vi "Convert Model.vi"(3 "error in (no error)":errorcluster, 4 "Model":string, 5 "Model Name In":T1) -> (0 "error out":errorcluster, 1 "SingleSource":bool, 2 "Model Name  Out":T1)   [LabVIEW 2018]
uses:
  Type Defs/Instrument Model.ctl
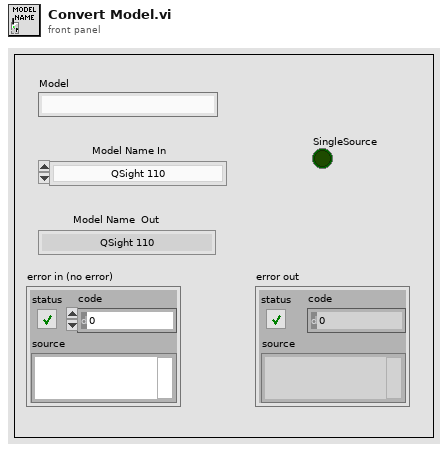
[diagram p1: front panel]
types:
  T1 = typedef "Instrument Model.ctl" = enum16{"QSight 110", "QSight 120", "QSight 210", "QSight 220", "QSight 410", "QSight 420", "IONICS 3Q 110", "IONICS 3Q 120", "IONICS 3Q 210", "IONICS 3Q 220", "IONICS 3Q 310", "IONICS 3Q 320", "Simulation (Single Source)", "Simulation (Dual Source)"}
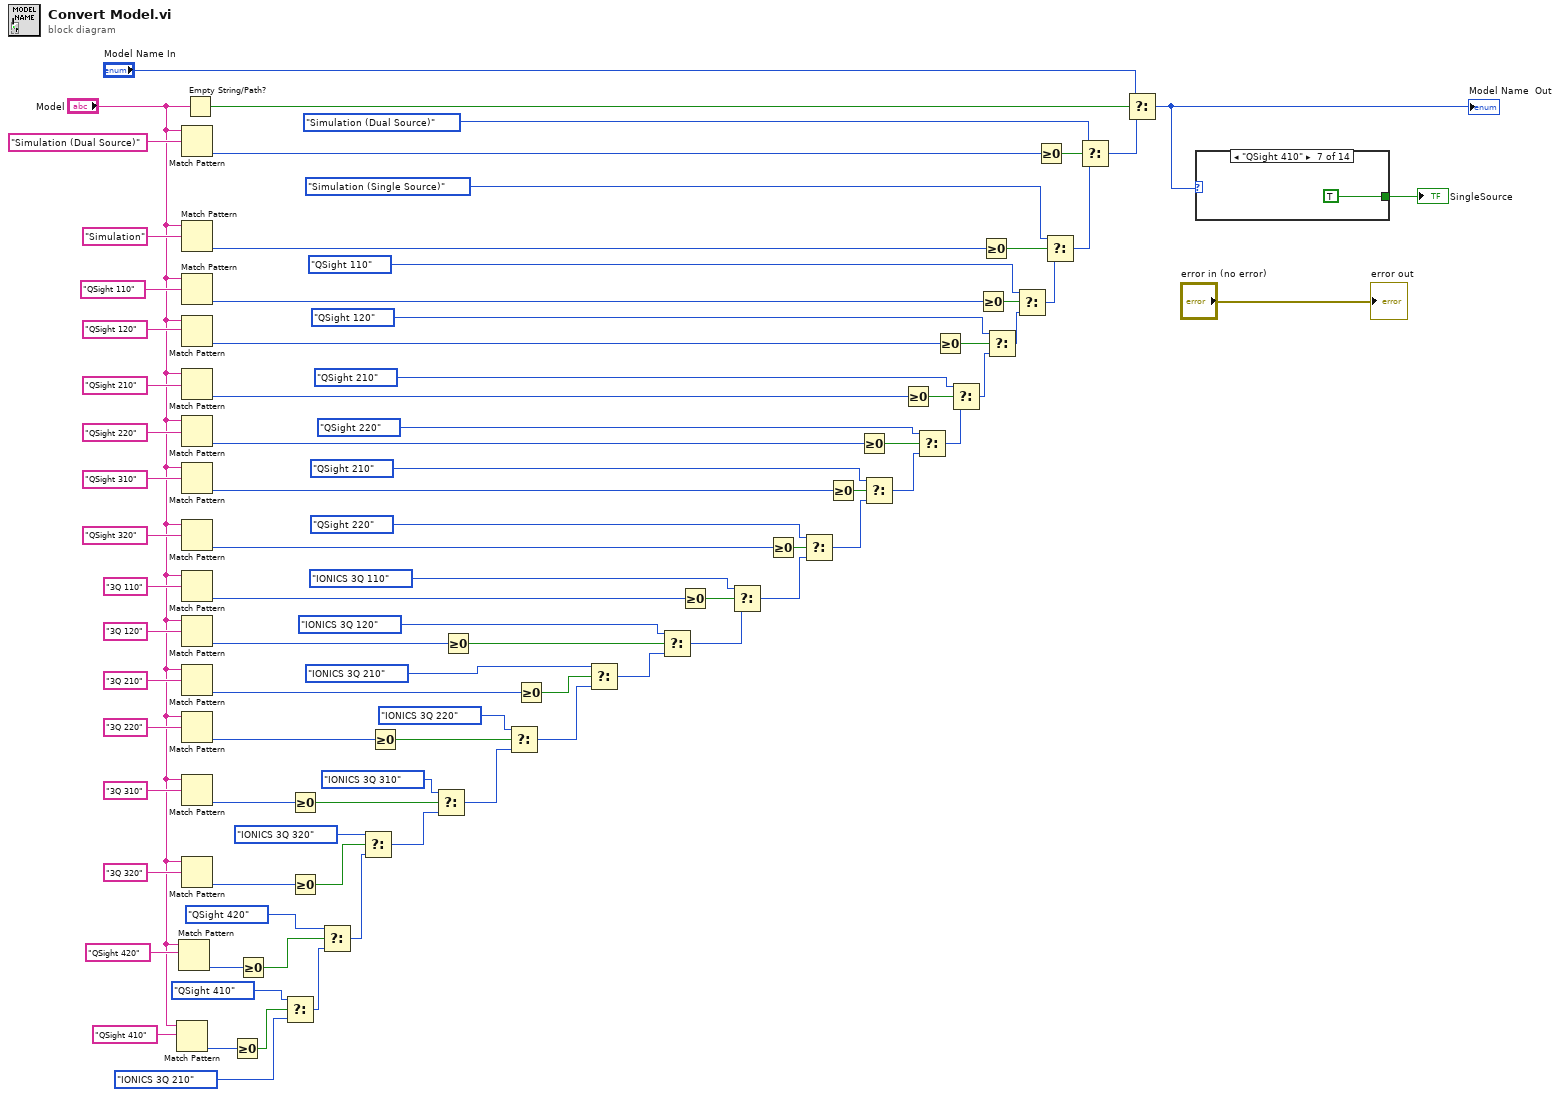
[diagram p0: block diagram]
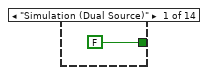
[diagram p2: hidden frame]
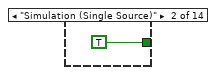
[diagram p3: hidden frame]
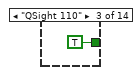
[diagram p4: hidden frame]
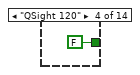
[diagram p5: hidden frame]
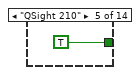
[diagram p6: hidden frame]
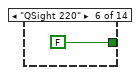
[diagram p7: hidden frame]
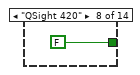
[diagram p8: hidden frame]
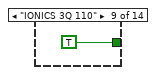
[diagram p9: hidden frame]
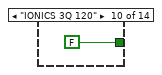
[diagram p10: hidden frame]
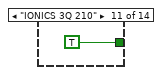
[diagram p11: hidden frame]
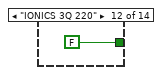
[diagram p12: hidden frame]
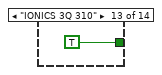
[diagram p13: hidden frame]
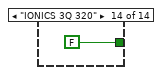
[diagram p14: hidden frame]
diagram:
  n1 = Match Pattern(string="Model", regular expression="QSight 410") -> (offset past match=w25:i32)  [unwired: 4 out]
  n2 = Match Pattern(string="Model", regular expression="QSight 420") -> (offset past match=w26:i32)  [unwired: 4 out]
  n3 = Match Pattern(string="Model", regular expression="Simulation (Dual Source)") -> (offset past match=w86:i32)  [unwired: 4 out]
  n4 = Match Pattern(string="Model", regular expression="Simulation") -> (offset past match=w74:i32)  [unwired: 4 out]
  n5 = Match Pattern(string="Model", regular expression="QSight 110") -> (offset past match=w44:i32)  [unwired: 4 out]
  n6 = Match Pattern(string="Model", regular expression="QSight 120") -> (offset past match=w45:i32)  [unwired: 4 out]
  n7 = Match Pattern(string="Model", regular expression="QSight 210") -> (offset past match=w79:i32)  [unwired: 4 out]
  n8 = Match Pattern(string="Model", regular expression="QSight 220") -> (offset past match=w80:i32)  [unwired: 4 out]
  n9 = Match Pattern(string="Model", regular expression="QSight 310") -> (offset past match=w32:i32)  [unwired: 4 out]
  n10 = Match Pattern(string="Model", regular expression="QSight 320") -> (offset past match=w36:i32)  [unwired: 4 out]
  n11 = Match Pattern(string="Model", regular expression="3Q 110") -> (offset past match=w72:i32)  [unwired: 4 out]
  n12 = Match Pattern(string="Model", regular expression="3Q 120") -> (offset past match=w73:i32)  [unwired: 4 out]
  n13 = Match Pattern(string="Model", regular expression="3Q 210") -> (offset past match=w65:i32)  [unwired: 4 out]
  n14 = Match Pattern(string="Model", regular expression="3Q 220") -> (offset past match=w50:i32)  [unwired: 4 out]
  n15 = Match Pattern(string="Model", regular expression="3Q 310") -> (offset past match=w53:i32)  [unwired: 4 out]
  n16 = Match Pattern(string="Model", regular expression="3Q 320") -> (offset past match=w54:i32)  [unwired: 4 out]
  n17 = Empty String/Path?(string/path="Model") -> (empty?=w59:bool)
  n18 = Greater Or Equal To 0?(x=w25) -> (x >= 0?=w23:bool)
  n19 = Greater Or Equal To 0?(x=w26) -> (x >= 0?=w24:bool)
  n20 = Select(t=Instrument_Model."QSight 410" ("Model Name"), s=w23, f=Instrument_Model."IONICS 3Q 210" ("Model Name")) -> (s? t:f=w21:T1)
  n21 = Greater Or Equal To 0?(x=w53) -> (x >= 0?=w52:bool)
  n22 = Greater Or Equal To 0?(x=w54) -> (x >= 0?=w55:bool)
  n23 = Select(t=Instrument_Model."QSight 420" ("Model Name"), s=w24, f=w21) -> (s? t:f=w22:T1)
  n24 = Select(t=Instrument_Model."IONICS 3Q 320" ("Model Name"), s=w55, f=w22) -> (s? t:f=w57:T1)
  n25 = Greater Or Equal To 0?(x=w50) -> (x >= 0?=w64:bool)
  n26 = Select(t=Instrument_Model."IONICS 3Q 310" ("Model Name"), s=w52, f=w57) -> (s? t:f=w49:T1)
  n27 = Greater Or Equal To 0?(x=w73) -> (x >= 0?=w70:bool)
  n28 = Select(t=Instrument_Model."IONICS 3Q 220" ("Model Name"), s=w64, f=w49) -> (s? t:f=w60:T1)
  n29 = Greater Or Equal To 0?(x=w65) -> (x >= 0?=w66:bool)
  n30 = Select(t=Instrument_Model."IONICS 3Q 210" ("Model Name"), s=w66, f=w60) -> (s? t:f=w61:T1)
  n31 = Select(t=Instrument_Model."IONICS 3Q 120" ("Model Name"), s=w70, f=w61) -> (s? t:f=w62:T1)
  n32 = Greater Or Equal To 0?(x=w72) -> (x >= 0?=w71:bool)
  n33 = Select(t=Instrument_Model."IONICS 3Q 110" ("Model Name"), s=w71, f=w62) -> (s? t:f=w34:T1)
  n34 = Greater Or Equal To 0?(x=w36) -> (x >= 0?=w37:bool)
  n35 = Select(t=Instrument_Model."QSight 220" ("Model Name"), s=w37, f=w34) -> (s? t:f=w31:T1)
  n36 = Greater Or Equal To 0?(x=w32) -> (x >= 0?=w33:bool)
  n37 = Greater Or Equal To 0?(x=w80) -> (x >= 0?=w81:bool)
  n38 = Select(t=Instrument_Model."QSight 210" ("Model Name"), s=w33, f=w31) -> (s? t:f=w30:T1)
  n39 = Greater Or Equal To 0?(x=w79) -> (x >= 0?=w78:bool)
  n40 = Select(t=Instrument_Model."QSight 220" ("Model Name"), s=w81, f=w30) -> (s? t:f=w84:T1)
  n41 = Greater Or Equal To 0?(x=w45) -> (x >= 0?=w42:bool)
  n42 = Select(t=Instrument_Model."QSight 210" ("Model Name"), s=w78, f=w84) -> (s? t:f=w41:T1)
  n43 = Greater Or Equal To 0?(x=w44) -> (x >= 0?=w43:bool)
  n44 = Greater Or Equal To 0?(x=w74) -> (x >= 0?=w75:bool)
  n45 = Select(t=Instrument_Model."QSight 120" ("Model Name"), s=w42, f=w41) -> (s? t:f=w40:T1)
  n46 = Select(t=Instrument_Model."QSight 110" ("Model Name"), s=w43, f=w40) -> (s? t:f=w39:T1)
  n47 = Greater Or Equal To 0?(x=w86) -> (x >= 0?=w85:bool)
  n48 = Select(t=Instrument_Model."Simulation (Single Source)" ("Model Name"), s=w75, f=w39) -> (s? t:f=w83:T1)
  n49 = Select(t=Instrument_Model."Simulation (Dual Source)" ("Model Name"), s=w85, f=w83) -> (s? t:f=w58:T1)
  n50 = Select(t="Model Name In", s=w59, f=w58) -> (s? t:f=w2:T1)
  "Model Name  Out" <- w2
  n51 = case shown="\"QSight 410\"" w2 {
    tunnel: [FALSE ("SingleSource") TRUE ("SingleSource") TRUE ("SingleSource") FALSE ("SingleSource") TRUE ("SingleSource") FALSE ("SingleSource") TRUE ("SingleSource") FALSE ("SingleSource") TRUE ("SingleSource") FALSE ("SingleSource") TRUE ("SingleSource") FALSE ("SingleSource") TRUE ("SingleSource") FALSE ("SingleSource")] -> w48
    frame "Simulation (Dual Source)" {
    }
    frame "Simulation (Single Source)" {
    }
    frame "QSight 110" {
    }
    frame "QSight 120" {
    }
    frame "QSight 210" {
    }
    frame "QSight 220" {
    }
    frame "QSight 410" {
    }
    frame "QSight 420" {
    }
    frame "IONICS 3Q 110" {
    }
    frame "IONICS 3Q 120" {
    }
    frame "IONICS 3Q 210" {
    }
    frame "IONICS 3Q 220" {
    }
    frame "IONICS 3Q 310" {
    }
    frame "IONICS 3Q 320" {
    }
  }
  "SingleSource" <- w48
  "error out" <- "error in (no error)"
